vi "DataTreeCtrlFM deleteData.vi"(8 "error in (no error)":errorcluster, 10 "deleteNames":string[](array[string]), 11 "TDMSAdv in":refnum<class "TDMSAdv.lvclass">) -> (0 "error out":errorcluster, 3 "TDMSAdv out":refnum<class "TDMSAdv.lvclass">)   [LabVIEW 2018, in "DataTreeCtrl.lvclass"]
uses:
  DataTreeCtrl.lvclass
  PublicSubVI/Class/FileManager/TDMSAdv.lvclass
  PublicSubVI/Class/FileManager/FM/ctl/_PC_Pub_FM fileReadFuncEnum.ctl
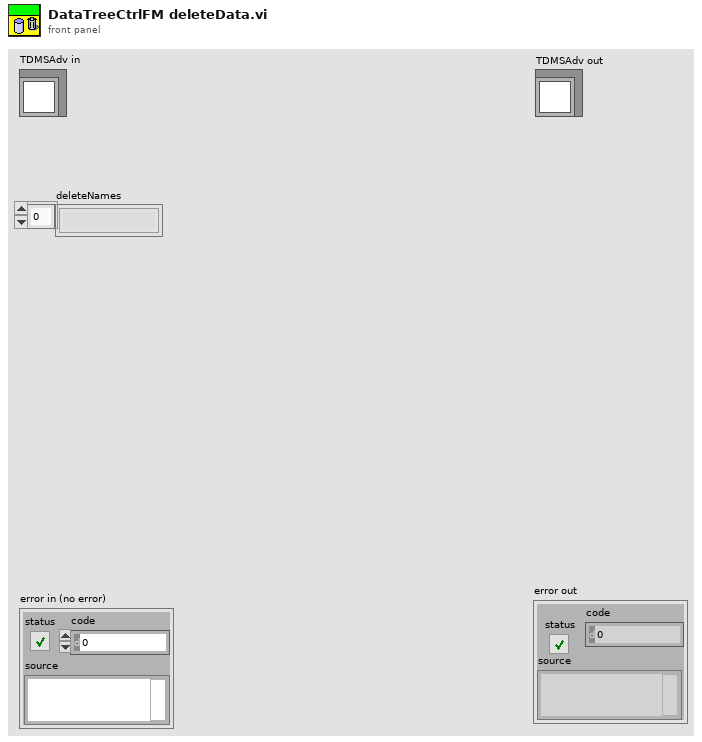
[diagram p1: front panel]
types:
  T1 = typedef "_PC_Pub_FM fileReadFuncEnum.ctl" = enum16{"getAllInfo", "getChromatogram", "getDataItems", "getTimeStamp", "getIdxData", "getIonization", "getRemark", "getAttrFormat"}
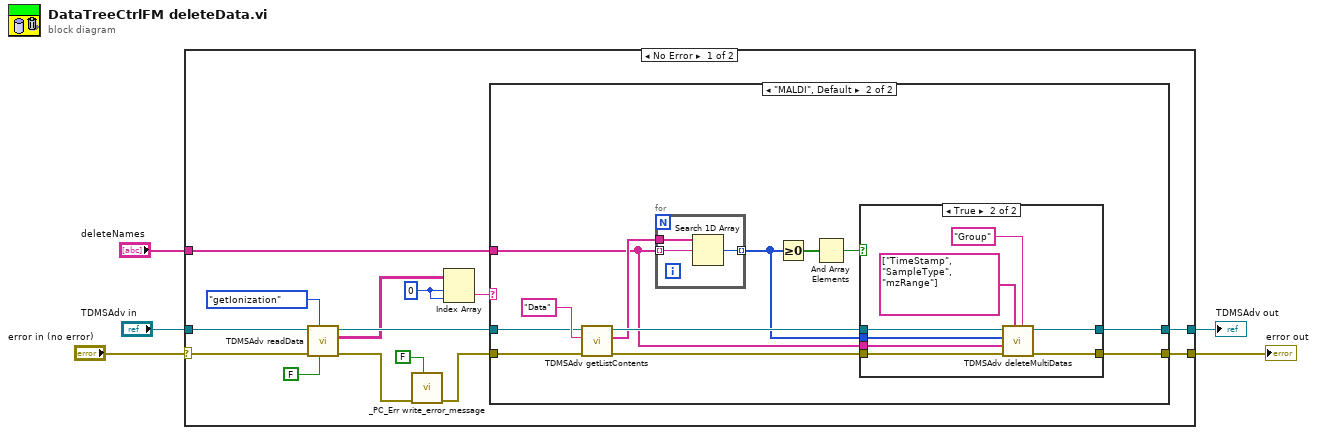
[diagram p0: block diagram]
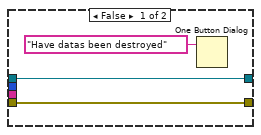
[diagram p3: hidden frame]
diagram:
  n1 = case shown="No Error" "error in (no error)" {
    selector: "error in (no error)" -> [w9 w49]
    tunnel: "deleteNames" -> [w19 _]
    tunnel: [w6 w49] -> w3
    tunnel: "TDMSAdv in" -> [w8 w48]
    tunnel: [w7 w48] -> w4
    frame No Error {
      w15 = 0 ("index (row)")
      n2 = call "TDMSAdv readData.vi"("stringSplit? (T)"=FALSE, "readEvent"=_PC_Pub_FM_fileReadFuncEnum."getIonization", "error in (no error)"=w9, "TDMSAdv in"=w8) -> ("error out"=w11:errorcluster, "outputArr"=w16:string[][], "TDMSAdv out"=w17:refnum<class "TDMSAdv.lvclass">)  [unwired: 4 in, 1 out]
      n3 = call "_PC_Err write_error_message.vi"("show msg( T )"=FALSE, "error in"=w11) -> ("error out"=w10:errorcluster)  [unwired: 9 in]
      n4 = Index Array(array=w16, index (row)=w15, index (col)=w15) -> (element=w14:string)
      n5 = case shown="\"MALDI\", Default" w14 {
        tunnel: [w21 w33] -> w7
        tunnel: [w20 w32] -> w6
        tunnel: w19 -> [_ w24]
        tunnel: w17 -> [w21 w27]
        tunnel: w10 -> [w20 w26]
        frame "False" {
        }
        frame "MALDI", Default {
          n6 = call "TDMSAdv getListContents.vi"("error in (no error)"=w26, "group name"="Data" ("group name in"), "TDMSAdv in"=w27) -> ("error out"=w30:errorcluster, "channels"=w28:string[], "TDMSAdv out"=w31:refnum<class "TDMSAdv.lvclass">)  [unwired: 6 in]
          n7 = for {
            tunnel: w28 -> [w47]
            tunnel: [w46] -> w25 mode=indexing
            tunnel: w24 -> [w45] mode=indexing
            n8 = Search 1D Array(1D array=w47, element=w45) -> (index of element=w46:i32)  [unwired: 1 in]
          }
          n9 = Greater Or Equal To 0?(x=w25) -> (x >= 0?=w23:bool[])
          n10 = And Array Elements(Boolean array=w23) -> (logical AND=w22:bool)
          n11 = case shown="True" w22 {
            tunnel: [w36 w44] -> w33
            tunnel: [w35 w43] -> w32
            tunnel: w31 -> [w36 w42]
            tunnel: w30 -> [w35 w41]
            tunnel: w25 -> [_ w40]
            tunnel: w24 -> [_ w39]
            frame False {
              n12 = One Button Dialog(message="Have datas been destroyed") -> ()  [unwired: 1 in, 1 out]
            }
            frame True {
              n13 = call "TDMSAdv deleteMultiDatas.vi"("group name"="Group", "channel names"=string[] ["TimeStamp", "SampleType", "mzRange"], "error in (no error)"=w41, "deleteNames"=w39, "deleteIndex"=w40, "TDMSAdv in"=w42) -> ("error out"=w43:errorcluster, "TDMSAdv out"=w44:refnum<class "TDMSAdv.lvclass">)  [unwired: 4 in]
            }
          }
        }
      }
    }
    frame Error {
    }
  }
  "TDMSAdv out" <- w4
  "error out" <- w3
